vi "N09_Array_For_Loop.vi"() -> ()   [LabVIEW 2023]
panel:
  out "x+y":dbl
  in  "Add Up to Index":i32
  in  "Array":dbl[](array[numeric])
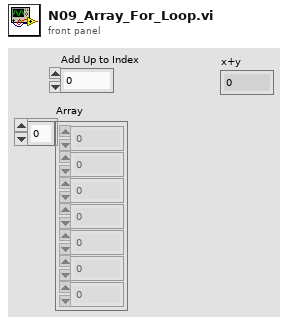
[diagram p1: front panel]
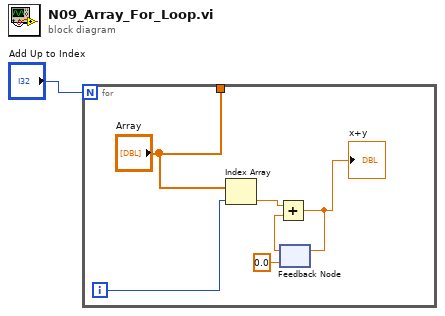
[diagram p0: block diagram]
diagram:
  n1 = for {
    N: "Add Up to Index" -> [_]
    tunnel: ["Array"] -> _
    i -> [w6]
    n2 = Index Array(array="Array", index=w6) -> (element=w5:dbl)
    n3 = feedback #1(0.0) -> (w3:dbl)
    n4 = Add(x=w5, y=w3) -> (x+y=w4:dbl)
    "x+y" <- w4
    n5 = feedback-in #1(w4) -> ()
  }
